vi "libssh2_channel_write_stderr.vi"(8 "error in (no error)":errorcluster, 10 "buffer":u8[](array[numeric]), 11 "channel":T1) -> (0 "error out":errorcluster, 3 "bytes written":i32)   [LabVIEW 2013, in "libssh2.lvlib"]
doc: "Write data to the standard error substream of a channel."
uses:
  libssh2.lvlib
  Channel Refnum.ctl
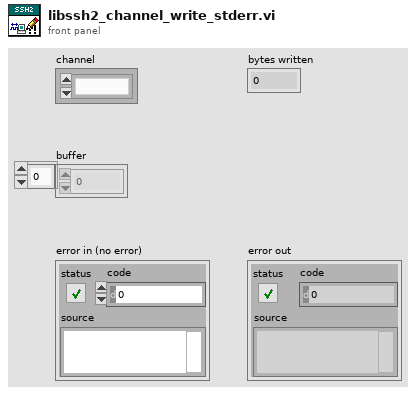
[diagram p1: front panel]
types:
  T1 = typedef "libssh2.lvlib/Channel Refnum.ctl" = refnum<k1>
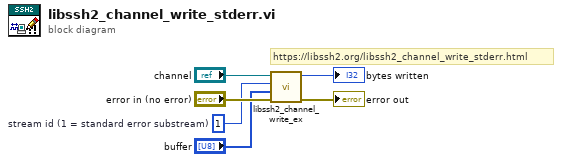
[diagram p0: block diagram]
diagram:
  w2 = 1  # stream id (1 = standard error substream)
  # "https://libssh2.org/libssh2_channel_write_stderr.html"
  n1 = call "libssh2_channel_write_ex.vi"("error in (no error)"="error in (no error)", "buffer"="buffer", "stream id"=w2, "channel"="channel") -> ("error out"=→"error out":errorcluster, "bytes written"=→"bytes written":i32)  [unwired: 6 in]
